vi "Delete Global Attribute.vi"(8 "Error In":errorcluster, 11 "Name":string) -> (0 "Error Out":errorcluster, 3 "dup Name":string)   [LabVIEW 2013, in "TS.lvlib"]
doc: "Non-reentrant."
uses:
  TS.lvlib
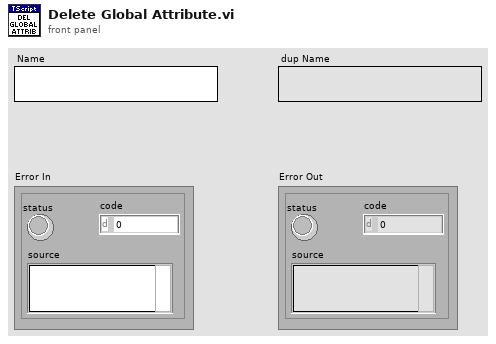
[diagram p1: front panel]
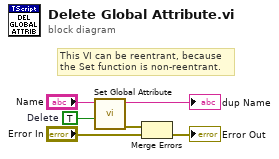
[diagram p0: block diagram]
diagram:
  w5 = TRUE  # Delete
  # "This VI can be reentrant, because\nthe Set function is non-reentrant."
  n1 = call "Set Global Attribute.vi"("Delete (F)"=w5, "Name"="Name") -> ("Error Out"=w2:errorcluster, "dup Name"=→"dup Name":string)  [unwired: 8 in]
  n2 = Merge Errors(w2, "Error In") -> (→"Error Out":errorcluster)
